vi "UnInitialize Owner Attribute.vi"(11 "Attribute.Owner":refnum<class "Attribute.Owner.lvclass">) -> ()   [LabVIEW 2021, in "smo.lvlib" / "Attribute.Owner.lvclass"]
uses:
  Attribute.Owner.lvclass
  Attribute.Owner.lvclass/Attribute.Owner.ctl
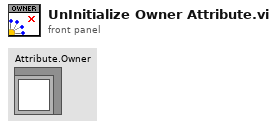
[diagram p1: front panel]
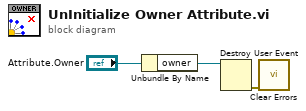
[diagram p0: block diagram]
diagram:
  n1 = Unbundle By Name("Attribute.Owner") -> ("owner"=w2:refnum<user-event>)
  n2 = Destroy User Event(user event=w2) -> (error out=w1:errorcluster)  [unwired: 1 in]
  n3 = call <vilib>:"Clear Errors.vi"("error in (no error)"=w1) -> ()  [unwired: 5 in, 2 out]
